vi "DAC Init Results.vi"(8 "error in":errorcluster, 9 "Log Details?":bool, 10 "tdms file":refnum<k34>, 11 "DAC TC Temperature in":refnum<class "DAC TC Temp DeepU.lvclass">) -> (0 "error out":errorcluster, 2 "tdms file out":refnum<k34>)   [LabVIEW 2019, in "DAC.lvlib" / "DAC TC Temp DeepU.lvclass"]
uses:
  DAC TC Temp DeepU.lvclass
  C:/Users/krio/Documents/LV_Projects/test-stand/App/DAC/DAC.lvclass
  DAC.lvclass/DAC.ctl
  DAC TC Temp DeepU.lvclass/DAC TC Temp DeepU.ctl
  DAC.lvclass
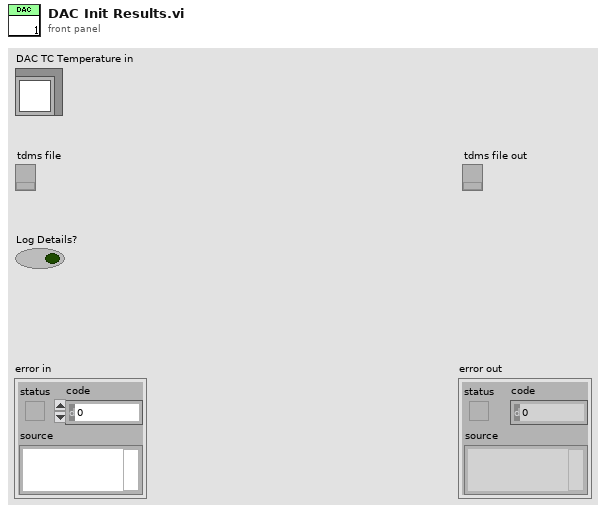
[diagram p1: front panel]
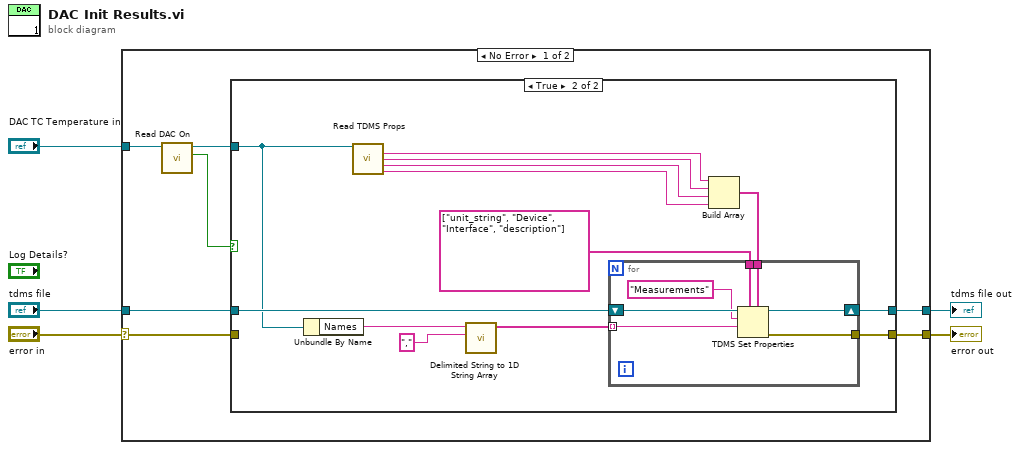
[diagram p0: block diagram]
diagram:
  n1 = case shown="No Error" "error in" {
    selector: "error in" -> [w7 w36]
    tunnel: [w10 w36] -> w2
    tunnel: "DAC TC Temperature in" -> [w9 _]
    tunnel: "tdms file" -> [w12 w35]
    tunnel: [w11 w35] -> w1
    frame No Error {
      n2 = call "Read DAC On.vi"("DAC in"=w9) -> ("DAC On"=w6:bool, "DAC out"=w8:refnum<class "DAC TC Temp DeepU.lvclass">)  [unwired: 8 in, 1 out]
      n3 = case shown="True" w6 {
        tunnel: w12 -> [w14 w27]
        tunnel: [w14 w26] -> w11
        tunnel: [w13 w25] -> w10
        tunnel: w8 -> [_ w19]
        tunnel: w7 -> [w13 _]
        frame False {
        }
        frame True {
          n4 = Unbundle By Name(w19) -> ("Names"=w22:string)
          n5 = call "Read TDMS Props.vi"("DAC in"=w19) -> ("Result Unit"=w18:string, "DAC Device"=w17:string, "DAC IO"=w16:string, "DAC Description"=w15:string)  [unwired: 10 in, 1 out]
          n6 = call <vilib>:"Delimited String to 1D String Array.vi"("delimiter"=",", "delimited string"=w22) -> ("string array"=w24:string[])  [unwired: 9 in]
          n7 = Build Array(w18, w17, w16, w15) -> (w21:string[])
          n8 = for {
            tunnel: w24 -> [w32] mode=indexing
            tunnel: string[] ["unit_string", "Device", "Interface", "description"] ("property names") -> [w31]
            tunnel: w21 -> [w30]
            tunnel: [w28] -> w25
            shift-right: [w29] -> w26
            shift-left: w27 -> [w34]
            n9 = TDMS Set Properties(5:w30, 7:w31, 9:w32, 10:"Measurements" ("group name in (Untitled)"), 11:w34) -> (0:w28:errorcluster, 3:w29:refnum<k34>)  [unwired: 1 in, 2 out]
          }
        }
      }
    }
    frame Error {
    }
  }
  "error out" <- w2
  "tdms file out" <- w1
